vi "开启试验判定.vi"(7 "Result":refnum<vi>, 10 "判定参数":T1={"手柄开启最大力"={"单位"="N", "下限"=3.0, "上限"=4.0}}, 11 "XY曲线":cluster{"X":dbl[], "Y":dbl[]}[](array[cluster])) -> (2 "判定项长度":i32, 3 "OK？":bool)   [LabVIEW 2020]
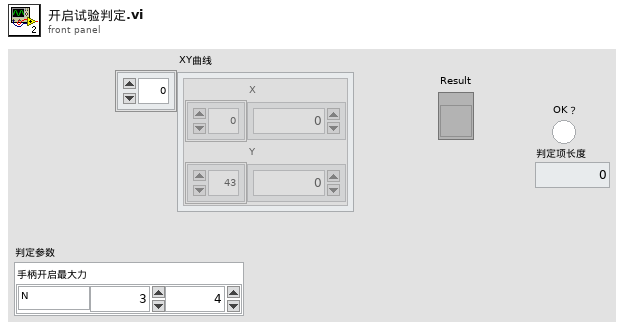
[diagram p1: front panel]
types:
  T1 = cluster{"手柄开启最大力":cluster{"单位":string, "下限":dbl, "上限":dbl}}
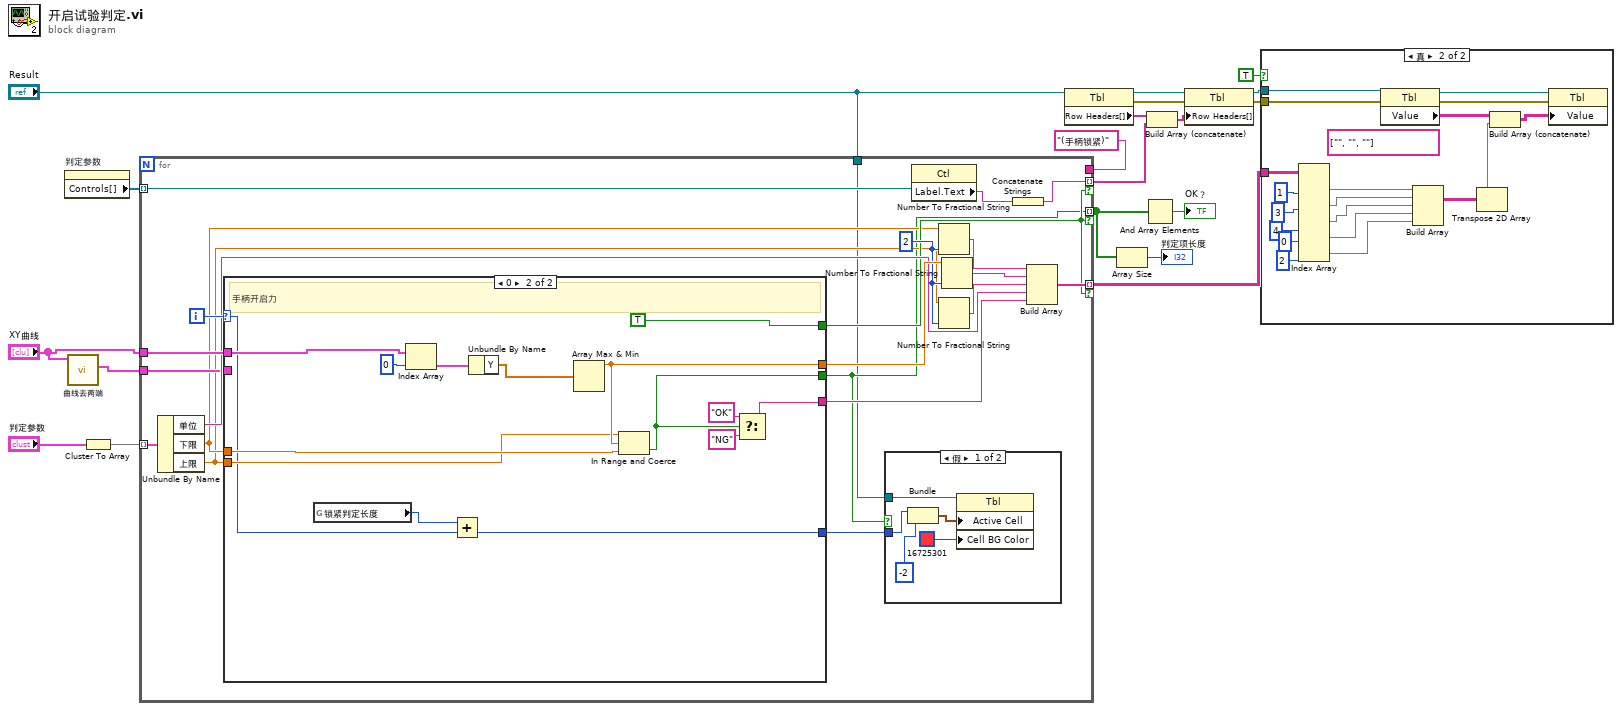
[diagram p0: block diagram]
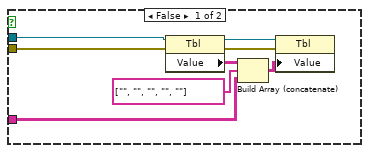
[diagram p2: hidden frame]
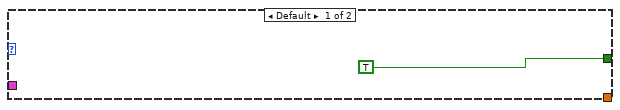
[diagram p4: hidden frame]
diagram:
  n1 = property on="判定参数" class="Clust (严格)"() -> ("Controls[]"=w11:refnum<vi>[])  [unwired: 2 in, 2 out]
  n2 = call "曲线去两端.vi"("曲线In"="XY曲线") -> ("启动曲线"=w6:cluster{"X":dbl[], "Y":dbl[]}[])  [unwired: 9 in, 1 out]
  n3 = Cluster To Array(cluster="判定参数") -> (array=w3:cluster{"单位":string, "下限":dbl, "上限":dbl}[])
  n4 = for {
    tunnel: w11 -> [w39] mode=indexing
    tunnel: "XY曲线" -> [w37]
    tunnel: [w22] -> w8 mode=indexing if=w28
    tunnel: [w30] -> w4 mode=indexing if=w28
    tunnel: [w24] -> w13 mode=indexing if=w28
    tunnel: w6 -> [w27]
    tunnel: "(手柄锁紧)" ("Label.Text") -> [_]
    tunnel: w3 -> [w23] mode=indexing
    tunnel: "Result" -> [w21]
    i -> [w40]
    w36 = i16 2 ("精度(6)")
    n5 = Unbundle By Name(w23) -> ("单位"=w31:string, "下限"=w26:dbl, "上限"=w25:dbl)
    n6 = case shown="0" w40 {
      selector: w40 -> [_ w49]
      tunnel: [_ w59] -> w38
      tunnel: w37 -> [_ w50]
      tunnel: [_ w56] -> w32
      tunnel: [_ w55] -> w22
      tunnel: w26 -> [_ w54]
      tunnel: w25 -> [_ w53]
      tunnel: [TRUE TRUE] -> w28
      tunnel: w27 -> [_ _]
      tunnel: [_ w48] -> w20
      frame Default {
      }
      frame 0 {
        # "手柄开启力"
        n7 = global read "判定参数.vi" "锁紧判定长度"() -> (w47:i32)
        n8 = Index Array(array=w50, index=0 ("索引")) -> (element=w60:cluster{"X":dbl[], "Y":dbl[]})
        n9 = Add(x=w47, y=w49) -> (x+y=w48:i32)
        n10 = Unbundle By Name(w60) -> ("Y"=w51:dbl[])
        n11 = Array Max & Min(array=w51) -> (max value=w59:dbl)  [unwired: 3 out]
        n12 = In Range and Coerce(upper limit=w53, x=w59, lower limit=w54) -> (In Range?=w55:bool)  [unwired: 1 out]
        n13 = Select(t="OK", s=w55, f="NG") -> (s? t:f=w56:string)
      }
    }
    n14 = case shown="假" w22 {
      tunnel: w21 -> [w45 _]
      tunnel: w20 -> [w43 _]
      frame False {
        n15 = Bundle(w43, "x"=-2) -> (w41:cluster{i32, "x":i32})  [unwired: 1 in]
        n16 = property class="Tbl"(reference=w45, "Active Cell"=w41, "Cell BG Color"=u32 16725301 ("活动单元格:单元格背景色")) -> ()  [unwired: 1 in, 2 out]
      }
      frame True {
      }
    }
    n17 = property class="Ctl"(reference=w39) -> ("Label.Text"=w29:string)  [unwired: 1 in, 2 out]
    n18 = Number To Fractional String(number=w26, precision (6)=w36) -> (F-format string=w35:string)  [unwired: 2 in]
    n19 = Number To Fractional String(number=w25, precision (6)=w36) -> (F-format string=w33:string)  [unwired: 2 in]
    n20 = Number To Fractional String(number=w38, precision (6)=w36) -> (F-format string=w34:string)  [unwired: 2 in]
    n21 = Concatenate Strings(w29) -> (w24:string)
    n22 = Build Array(w35, w34, w33, w31, w32) -> (w30:string[])
  }
  n23 = property class="Tbl"(reference="Result") -> (reference out=w15:refnum<vi>, error out=w18:errorcluster, "Row Headers[]"=w12:string[])  [unwired: 1 in]
  n24 = Array Size(array=w8) -> (size(s)=→"判定项长度":i32)
  n25 = And Array Elements(Boolean array=w8) -> (logical AND=→"OK？":bool)
  n26 = Build Array (concatenate)(w12, w13) -> (w14:string[])
  n27 = property class="Tbl"(reference=w15, error in=w18, "Row Headers[]"=w14) -> (reference out=w16:refnum<vi>, error out=w17:errorcluster)
  n28 = case shown="真" TRUE {
    tunnel: w17 -> [w67 w87]
    tunnel: w16 -> [w64 w84]
    tunnel: w4 -> [w63 w81]
    frame False {
      n29 = property class="Tbl"(reference=w64, error in=w67) -> (reference out=w65:refnum<vi>, error out=w66:errorcluster, "Value"=w68:string[][])
      n30 = Build Array (concatenate)(w68, string[] ["", "", "", "", ""], w63) -> (w69:string[][])
      n31 = property class="Tbl"(reference=w65, error in=w66, "Value"=w69) -> ()  [unwired: 2 out]
    }
    frame True {
      (unwired) string[] ["", "", ""]
      n32 = Index Array(array=w81, index (col) #1=1 ("禁用的索引 (列)"), index (col) #2=3 ("索引 (列)"), index (col) #3=4 ("索引 (列)"), index (col) #4=0 ("索引 (列)"), index (col) #5=2 ("索引 (列)")) -> (element #1=w76:string[], element #2=w75:string[], element #3=w74:string[], element #4=w73:string[], element #5=w72:string[])  [unwired: 5 in]
      n33 = property class="Tbl"(reference=w84, error in=w87) -> (reference out=w85:refnum<vi>, error out=w86:errorcluster, "Value"=w88:string[][])
      n34 = Build Array(w76, w75, w74, w73, w72) -> (w78:string[][])
      n35 = Transpose 2D Array ("二维数组转置")(2D array=w78) -> (transposed array=w70:string[][])
      n36 = Build Array (concatenate)(w88, w70) -> (w77:string[][])
      n37 = property class="Tbl"(reference=w85, error in=w86, "Value"=w77) -> ()  [unwired: 2 out]
    }
  }
